vi "Main.vi"() -> ()   [LabVIEW 2017]
doc: "Use this template to build a user interface event handler design pattern. Use this pattern for dialog boxes and other user interfaces. You also can create and execute user-defined events that the VI can handle the same way as user interface events."
uses:
  <vilib>/Utility/NIReport.llb/HTML Report Image Alignment.ctl
  <vilib>/Utility/NIReport.llb/image depth.ctl
  <vilib>/addons/database/Connection.llb/DB Tools Open Connec (Path).vi
  <vilib>/addons/database/Auxilliary.llb/DB Tools Format Datetime String (Time Stamp).vi
  GLOBAL/auto.vi
  <vilib>/Utility/NIReport.llb/Append Report Text (str wrap).vi
  <vilib>/Utility/NIReport.llb/NI_report.lvclass
  <vilib>/addons/database/NI_Database_API.lvlib
  <vilib>/Utility/NIReport.llb/NI_ReportGenerationCore.lvlib
panel:
  out "resulting string":path
  in  "import state 3":bool
  out "User Name":string
  out "time taken in sec":dbl
  out "Peak_valley_point":ext[](array[numeric])
  out "data size":i32
  out "A*C":bool
  out "L/Min":bool
  out "BAR":bool
  out "Min Peak/Min":dbl
  out "Max Valley/Min":dbl
  out "Status bar":string
  in  "import state 2":bool
  out "SELECTED RECIPE":string
  out "BARCODE_FOUND":bool
  out "DB CONN":bool
  in  "Graph":bool
  out "table":string[][](table)
  out "GRAPH":cluster{timestamp[], ext[]}[](graph)
  out "TEST RESULT":bool
  in  "BARCODE":string
  out "SELECTED FILE PATH":path
  in  "Import File":bool
  in  "SELECT MEASURED FILE":i32(listbox)
  out "error out":errorcluster
  in  "File Name":string
  in  "Report Files Folder":path
  in  "Convert":bool
  in  "BROWSE FILE FOLDER":path
  in  "stop":bool
  # "Main"
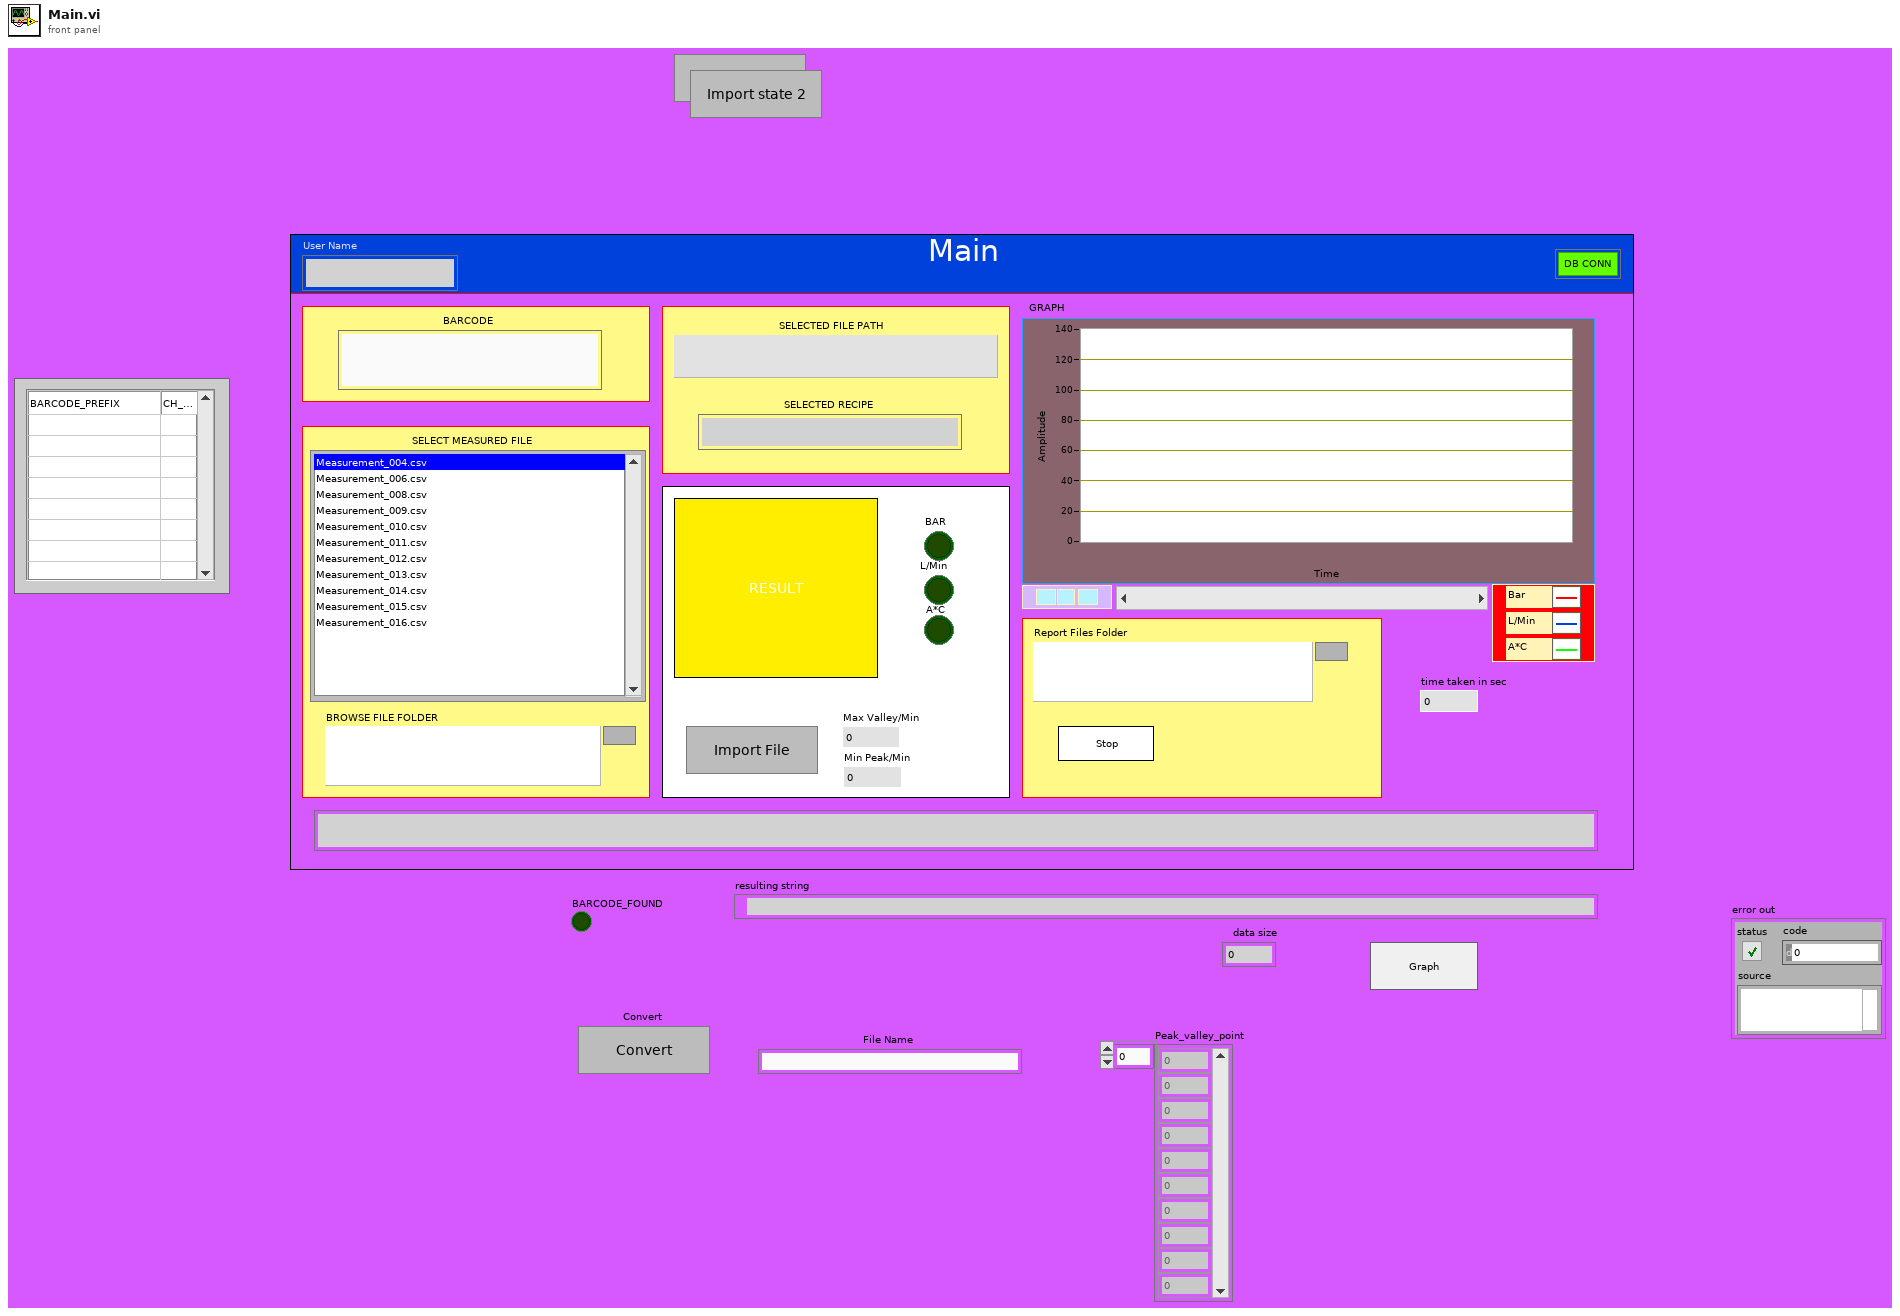
[diagram p1: front panel]
types:
  T1 = cluster{"Files":string[], "Browse File":path, "TIMEOUT":i32, "GRAPH":cluster{timestamp[], ext[]}[], "CHL 1":cluster{"chl1 MIN":dbl, "chl1 MAX":dbl, "chl1 thrshold":dbl}, "CHL 2":cluster{"chl2 MIN":dbl, "chl2 MAX":dbl, "chl2 thrshold":dbl}, "CHL 3":cluster{"chl3 MIN":dbl, "chl3 MAX":dbl, "chl3 thrshold":dbl}, "Report File":path, "Data_to_report":cluster{"date/time string":string, "User Name":string, "BARCODE":string, "SELECTED RECIPE":string, "Rst":string}}
  T2 = typedef "NI_Database_API.lvlib/Conn ObjectReference.ctl" = refnum<k1>
  T3 = enum32{"Invalid", "Standard", "Closed", "Hidden", "Minimized", "Maximized"}
  T4 = cluster{"position (excel)":cluster{"row":i32, "column":i32}, "name (excel)":string, "bookmark (word)":string}
  T5 = cluster{"position (Excel)":cluster{"row":i32, "column":i32}, "name (Excel)":string, "bookmark (Word)":string}
  T6 = typedef "NI_ReportGenerationCore.lvlib/HTML Report Image Alignment.ctl" = enum16{"(default)", "LEFT", "RIGHT", "TOP", "TEXTTOP", "MIDDLE", "ABSMIDDLE", "BASELINE", "BOTTOM", "ABSBOTTOM"}
  T7 = enum16{"Standard Report", "HTML", "Word", "Excel"}
  T8 = enum16{"maximized", "minimized", "normal", "no change"}
  T9 = cluster{"chl2 MIN":dbl, "chl2 MAX":dbl, "chl2 thrshold":dbl}
  T10 = cluster{"chl1 MIN":dbl, "chl1 MAX":dbl, "chl1 thrshold":dbl}
  T11 = cluster{"chl3 MIN":dbl, "chl3 MAX":dbl, "chl3 thrshold":dbl}
  T12 = cluster{"date/time string":string, "User Name":string, "BARCODE":string, "SELECTED RECIPE":string, "Rst":string}
  T13 = typedef "NI_ReportGenerationCore.lvlib/image depth.ctl" = u16
  T14 = enum32{"invalid app kind", "Development System", "Run Time System", "Student Edition", "Embedded LabVIEW", "Evaluation", "Custom"}
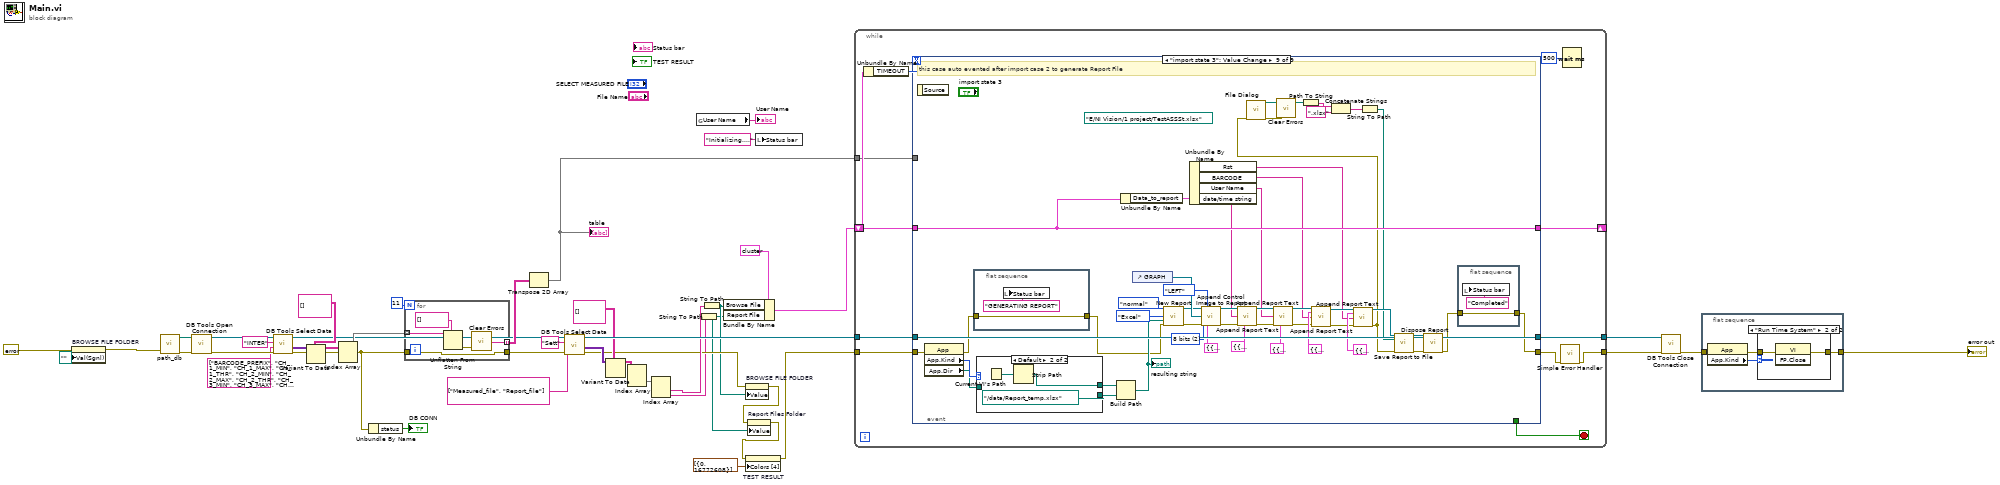
[diagram p0: block diagram]
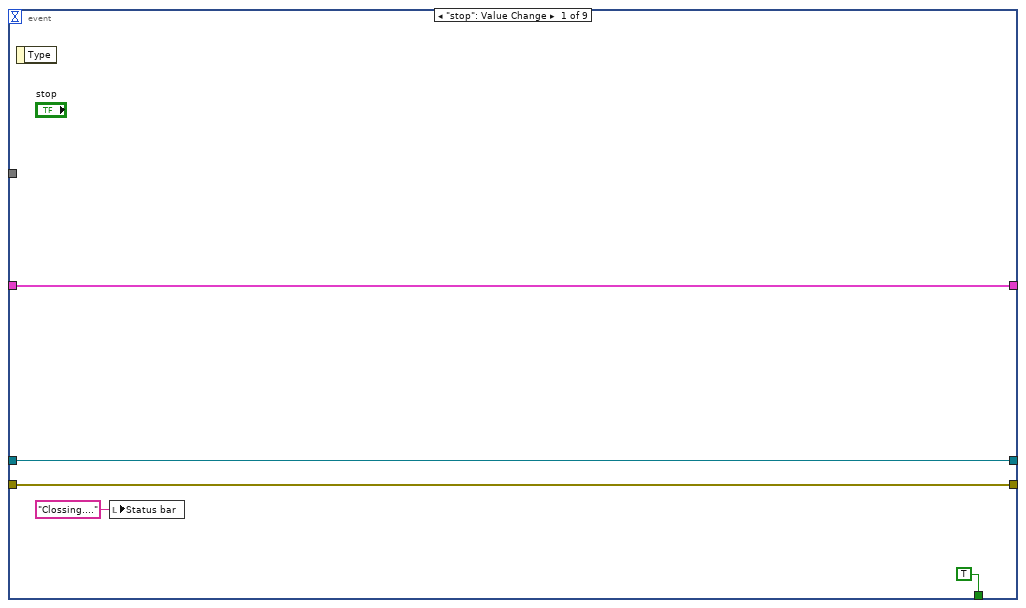
[diagram p3: hidden frame]
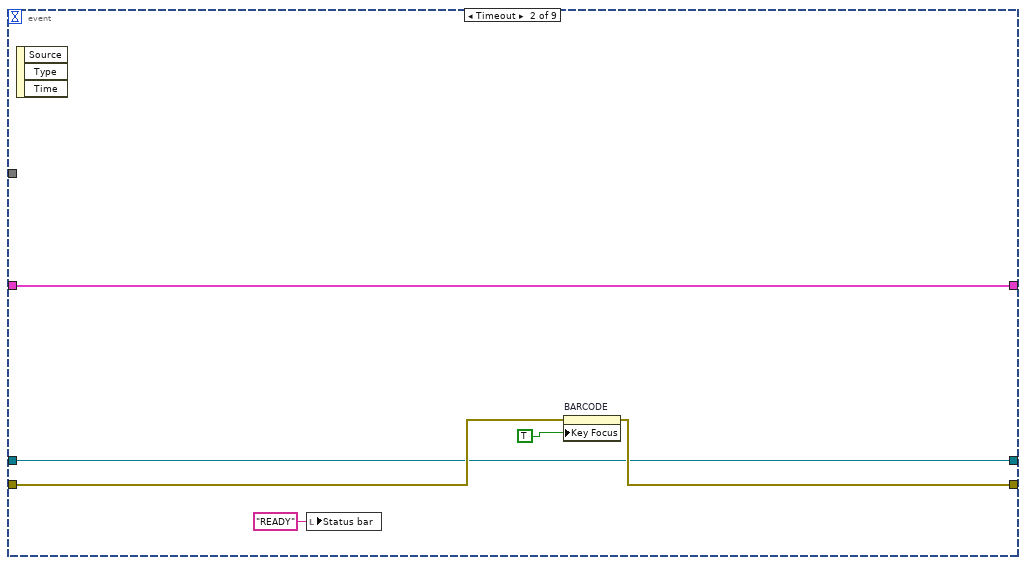
[diagram p4: hidden frame]
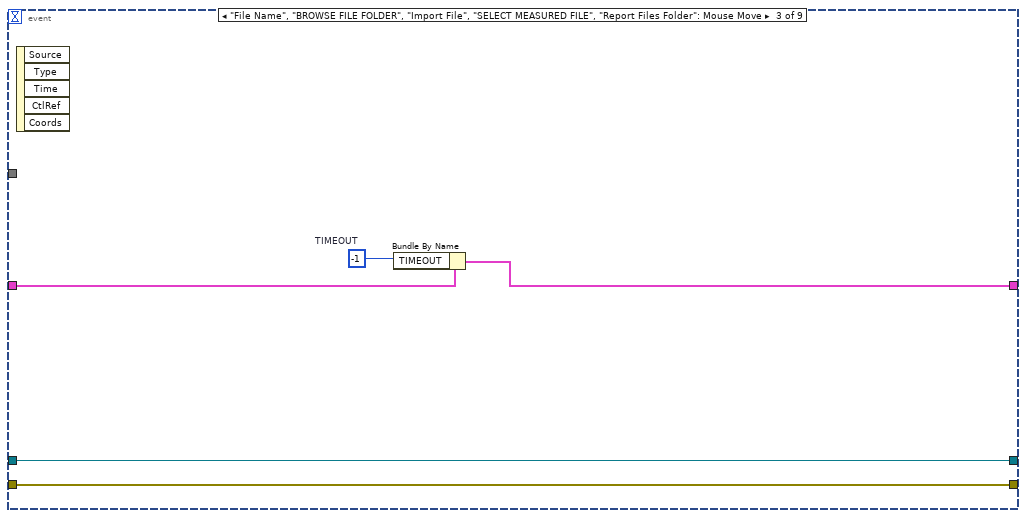
[diagram p5: hidden frame]
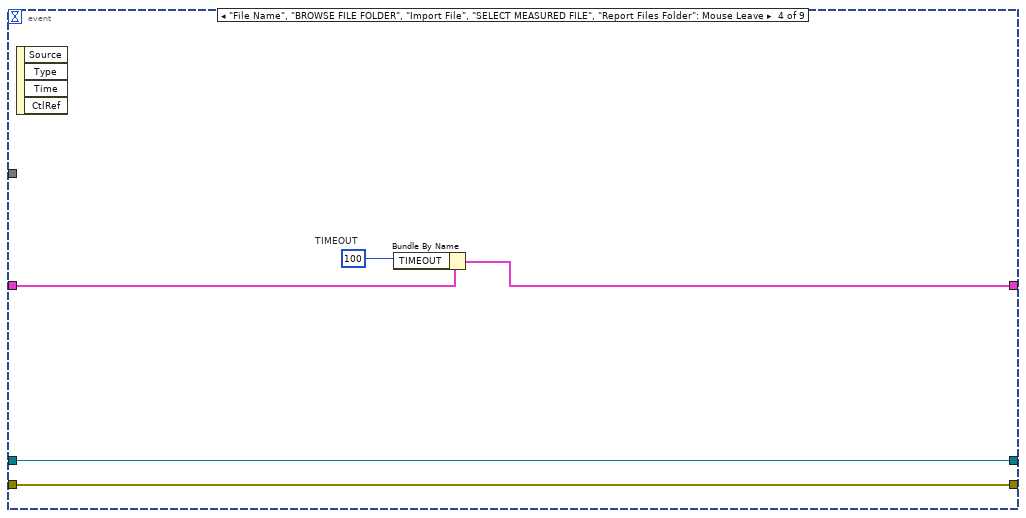
[diagram p6: hidden frame]
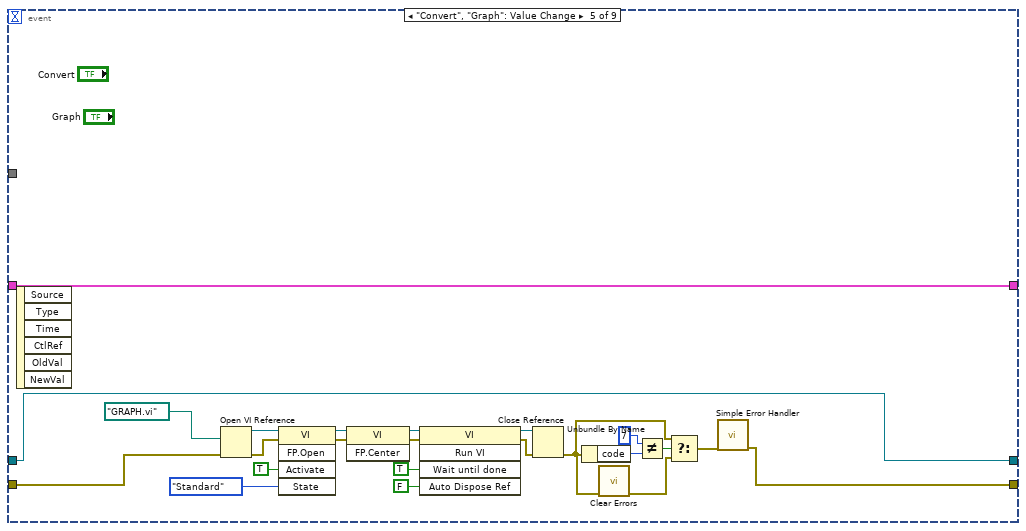
[diagram p7: hidden frame]
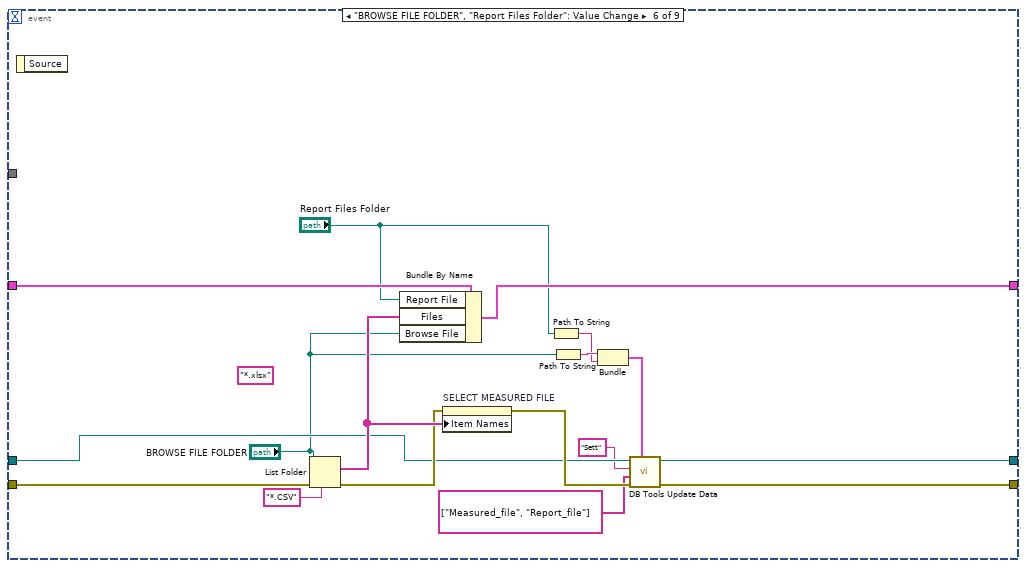
[diagram p8: hidden frame]
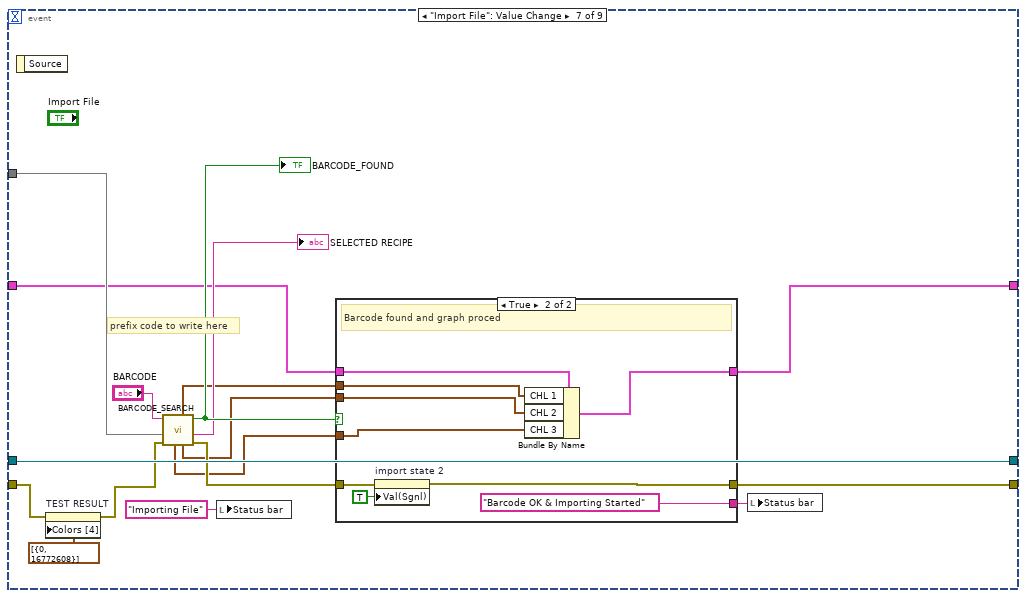
[diagram p9: hidden frame]
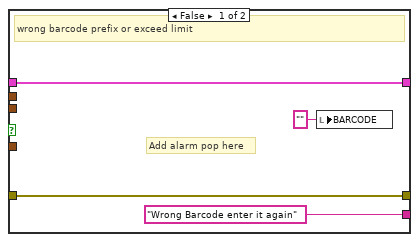
[diagram p10: hidden frame]
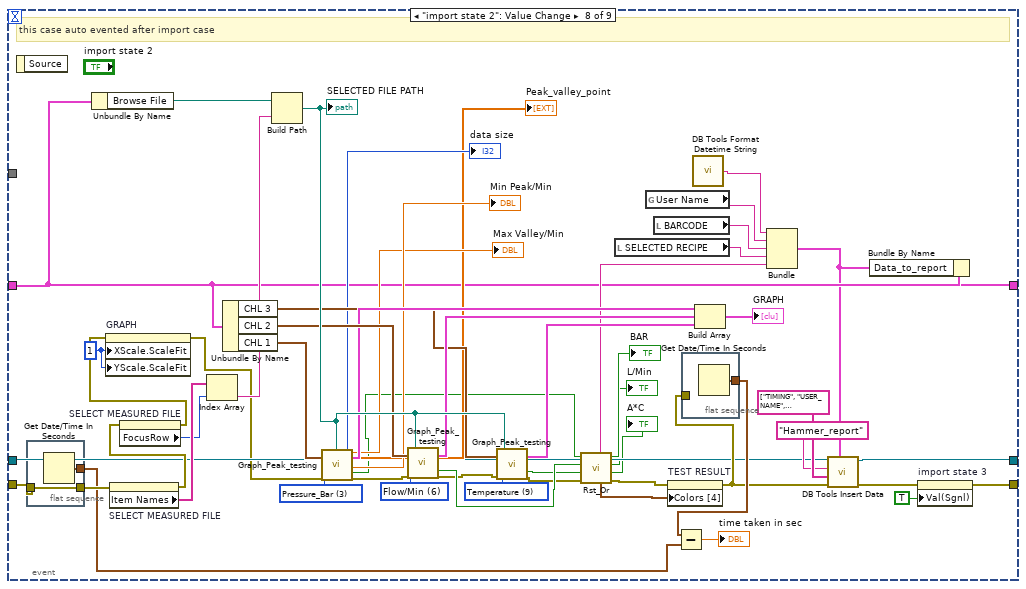
[diagram p11: hidden frame]
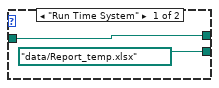
[diagram p12: hidden frame]
diagram:
  n1 = property on="BROWSE FILE FOLDER" class="Path"(error in=errorcluster {"status"=FALSE, "code"=0, "source"=""} ("error out 2"), "Val(Sgnl)"=path "" ("BROWSE FILE FOLDER")) -> (error out=w13:errorcluster)  [unwired: 1 in, 1 out]
  n2 = call "path_db.vi"("error in"=w13) -> ("error out"=w38:errorcluster, "resulting string"=w37:path)  [unwired: 9 in]
  n3 = call-poly <vilib>:"DB Tools Open Connection.vi"("error in (no error)"=w38, "connection information"=w37) -> ("error out"=w43:errorcluster, "connection reference"=w44:T2)  [unwired: 6 in]
  n4 = call <vilib>:"DB Tools Select Data.vi"("error in (no error)"=w43, "columns"=string[] ["BARCODE_PREFIX", "CH_1_MIN", "CH_1_MAX", "CH_1_THR", "CH_2_MIN", "CH_2_MAX", "CH_2_THR", "CH_3_MIN", "CH_3_MAX", "CH_3_THR", "RECIPE_NAME"], "table"="INTER", "connection reference"=w44) -> ("error out"=w31:errorcluster, "data"=w40:variant[][], "connection reference out"=w26:T2)  [unwired: 2 in]
  n5 = Variant To Data(type=string[][] [], Variant=w40) -> (data=w39:string[][])  [unwired: 1 in, 1 out]
  n6 = Index Array(array=w39) -> (element=w34:string[])  [unwired: 2 in]
  n7 = Unbundle By Name(w31) -> ("status"=→"DB CONN":bool)
  n8 = for {
    N: 11 -> [_]
    tunnel: w34 -> [w48] mode=indexing
    tunnel: [w46] -> w33 mode=indexing
    tunnel: w31 -> [w45]
    tunnel: [w45] -> w27
    n9 = Unflatten From String(type=string[] [], binary string=w48) -> (value=w46:string[], error out=w49:errorcluster)  [unwired: 3 in, 1 out]
    n10 = call <vilib>:"Clear Errors.vi"("error in (no error)"=w49) -> ()  [unwired: 5 in, 2 out]
  }
  n11 = Transpose 2D Array(2D array=w33) -> (transposed array=w11:string[][])
  "table" <- w11
  n12 = call <vilib>:"DB Tools Select Data.vi"("error in (no error)"=w27, "columns"=string[] ["Measured_file", "Report_file"], "table"="Sett", "connection reference"=w26) -> ("error out"=w16:errorcluster, "data"=w24:variant[][], "connection reference out"=w25:T2)  [unwired: 2 in]
  n13 = Variant To Data(type=string[][] [], Variant=w24) -> (data=w22:string[][])  [unwired: 1 in, 1 out]
  n14 = Index Array(array=w22) -> (element=w18:string[])  [unwired: 2 in]
  n15 = Index Array(array=w18) -> (element #1=w17:string, element #2=w10:string)  [unwired: 2 in]
  n16 = global read "auto.vi" "User Name"() -> (→"User Name":string)
  n17 = String To Path(string=w10) -> (path=w9:path)
  n18 = String To Path(string=w17) -> (path=w15:path)
  n19 = Bundle By Name(cluster=T1 {"Files"=[], "Browse File"=path "", "TIMEOUT"=100, "GRAPH"=[{array[68443 elements], array[68443 elements]}, {array[68363 elements], array[68363 elements]}, {array[40500 elements], array[40500 elements]}], "CHL 1"={"chl1 MIN"=110.0, "chl1 MAX"=130.0, "chl1 thrshold"=120.0}, "CHL 2"={"chl2 MIN"=33.0, "chl2 MAX"=35.0, "chl2 thrshold"=25.0}, "CHL 3"={"chl3 MIN"=20.0, "chl3 MAX"=30.0, "chl3 thrshold"=34.0}, "Report File"=path "", "Data_to_report"={"date/time string"="", "User Name"="", "BARCODE"="", "SELECTED RECIPE"="", "Rst"=""}}, "Browse File"=w15, "Report File"=w9) -> (w19:T1)
  n20 = property on="BROWSE FILE FOLDER" class="Path"(error in=w16, "Value"=w15) -> (error out=w8:errorcluster)  [unwired: 1 in, 1 out]
  n21 = property on="Report Files Folder" class="Path"(error in=w8, "Value"=w9) -> (error out=w7:errorcluster)  [unwired: 1 in, 1 out]
  n22 = property on="TEST RESULT" class="Bool"(error in=w7, "Colors [4]"=cluster{u32, u32}[] [{0, 16772608}]) -> (error out=w1:errorcluster)  [unwired: 1 in, 1 out]
  n23 = local write "Status bar"("Initializing...." ("Status bar")) -> ()
  n24 = while {
    tunnel: w1 -> [w58]
    tunnel: [w50] -> w30
    shift-right: [w57] -> _
    shift-left: w19 -> [w55]
    tunnel: w25 -> [w53]
    tunnel: [w54] -> w29
    tunnel: w11 -> [w52]
    stop <- w60 stop-if-true
    n25 = Unbundle By Name(w55) -> ("TIMEOUT"=w56:i32)
    n26 = event shown="[8] \"import state 3\": Value Change" {
      selector: _ -> [_ _ _ _ _ _ _ _ _]
      dyn-events: _ -> [_ _ _ _ _ _ _ _ _]
      timeout: w56 -> [_ _ _ _ _ _ _ _ _]
      tunnel: [TRUE _ _ _ _ _ _ _ _] -> w60
      tunnel: w58 -> [w64 w69 w76 w81 w84 w121 w125 w187 w251]
      tunnel: [w64 w68 w76 w81 w83 w114 w135 w162 w218] -> w51
      tunnel: w55 -> [w65 w71 w75 w80 w104 w120 w131 w160 w239]
      tunnel: [w65 w71 w74 w79 w104 w119 w130 w159 w239] -> w57
      tunnel: [w62 w67 w72 w77 w82 w112 w138 w178 w256] -> w54
      tunnel: w53 -> [w62 w67 w72 w77 w82 w113 w138 w179 w256]
      tunnel: w52 -> [_ _ _ _ _ _ w132 _ _]
      event "stop": Value Change {
        n27 = event-data() -> ()  [unwired: 1 in, 1 out]
        n28 = local write "Status bar"("Clossing...." ("Status bar")) -> ()
      }
      event Timeout {
        n29 = event-data() -> ()  [unwired: 1 in, 3 out]
        n30 = local write "Status bar"("READY" ("Status bar")) -> ()
        n31 = property on="BARCODE" class="Str"(error in=w69, "Key Focus"=TRUE) -> (error out=w68:errorcluster)  [unwired: 1 in, 1 out]
      }
      event "File Name", "BROWSE FILE FOLDER", "Import File", "SELECT MEASURED FILE", "Report Files Folder": Mouse Move {
        w73 = -1  # TIMEOUT
        n32 = event-data() -> ()  [unwired: 1 in, 5 out]
        n33 = Bundle By Name(cluster=w75, "TIMEOUT"=w73) -> (w74:T1)
      }
      event "File Name", "BROWSE FILE FOLDER", "Import File", "SELECT MEASURED FILE", "Report Files Folder": Mouse Leave {
        w78 = 100  # TIMEOUT
        n34 = event-data() -> ()  [unwired: 1 in, 4 out]
        n35 = Bundle By Name(cluster=w80, "TIMEOUT"=w78) -> (w79:T1)
      }
      event "Convert", "Graph": Value Change {
        n36 = event-data() -> ()  [unwired: 1 in, 6 out]
        n37 = Open VI Reference(vi path=path "GRAPH.vi", error in (no error)=w84) -> (vi reference=w91:refnum<vi>, error out=w103:errorcluster)  [unwired: 4 in]
        n38 = invoke class="VI" method="FP.Open"(reference=w91, error in=w103, "Activate"=TRUE ("Activate?"), "State"=T3."Standard") -> (reference out=w102:refnum<vi>, error out=w97:errorcluster)  [unwired: 1 in, 3 out]
        n39 = invoke class="VI" method="FP.Center"(reference=w102, error in=w97) -> (reference out=w98:refnum<vi>, error out=w99:errorcluster)  [unwired: 1 in, 1 out]
        n40 = invoke class="VI" method="Run VI"(reference=w98, error in=w99, "Wait until done"=TRUE ("Wait Until Done"), "Auto Dispose Ref"=FALSE ("Auto Dispose Reference")) -> (reference out=w100:refnum<vi>, error out=w101:errorcluster)  [unwired: 1 in, 3 out]
        n41 = Close Reference(reference=w100, error in (no error)=w101) -> (error out=w92:errorcluster)
        n42 = Unbundle By Name(w92) -> ("code"=w96:i32)
        n43 = call <vilib>:"Clear Errors.vi"("error in (no error)"=w92) -> ("error out"=w94:errorcluster)  [unwired: 5 in, 1 out]
        n44 = Not Equal?(x=7, y=w96) -> (x != y?=w95:bool)
        n45 = Select(t=w92, s=w95, f=w94) -> (s? t:f=w93:errorcluster)
        n46 = call <vilib>:"Simple Error Handler.vi"("error in (no error)"=w93) -> ("error out"=w83:errorcluster)  [unwired: 4 in, 4 out]
      }
      event "BROWSE FILE FOLDER", "Report Files Folder": Value Change {
        (unwired) "*.xlsx" ("pattern")
        n47 = event-data() -> ()  [unwired: 1 in, 1 out]
        n48 = List Folder(path="BROWSE FILE FOLDER", pattern="*.CSV", error in=w121) -> (filenames=w117:string[], error out=w116:errorcluster)  [unwired: 1 in, 2 out]
        n49 = Bundle By Name(cluster=w120, "Report File"="Report Files Folder", "Files"=w117, "Browse File"="BROWSE FILE FOLDER") -> (w119:T1)
        n50 = property on="SELECT MEASURED FILE" class="LstBox (strict)"(error in=w116, "Item Names"=w117) -> (error out=w115:errorcluster)  [unwired: 1 in, 1 out]
        n51 = Path To String(path="Report Files Folder") -> (string=w106:string)
        n52 = Path To String(path="BROWSE FILE FOLDER") -> (string=w108:string)
        n53 = Bundle(w108, w106) -> (w111:cluster{string, string})  [unwired: 1 in]
        n54 = call <vilib>:"DB Tools Update Data.vi"("data"=w111, "error in (no error)"=w115, "columns"=string[] ["Measured_file", "Report_file"], "table"="Sett", "connection reference"=w113) -> ("error out"=w114:errorcluster, "connection reference out"=w112:T2)  [unwired: 5 in]
      }
      event "Import File": Value Change {
        # "prefix code to write here"
        n55 = event-data() -> ()  [unwired: 1 in, 1 out]
        n56 = property on="TEST RESULT" class="Bool"(error in=w125, "Colors [4]"=cluster{u32, u32}[] [{0, 16772608}]) -> (error out=w124:errorcluster)  [unwired: 1 in, 1 out]
        n57 = call "BARCODE_SEARCH.vi"("error in"=w124, "BARCODE_TABLE"=w132, "BARCODE_TO_SEARCH"="BARCODE") -> ("error out"=w136:errorcluster, "Recipe name"=→"SELECTED RECIPE":string, "BARCODE_FOUND"=w134:bool, "CHL 2"=w128:T9, "CHL 1"=w129:T10, "CHL 3"=w127:T11)  [unwired: 2 in, 1 out]
        "BARCODE_FOUND" <- w134
        n58 = local write "Status bar"("Importing File" ("Status bar")) -> ()
        n59 = case shown="True" w134 {
          tunnel: [w142 w149] -> w135
          tunnel: w136 -> [w142 w150]
          tunnel: [w141 w147] -> w130
          tunnel: w131 -> [w141 w148]
          tunnel: w129 -> [_ w146]
          tunnel: w128 -> [_ w145]
          tunnel: w127 -> [_ w144]
          tunnel: ["Wrong Barcode enter it again" ("Status bar") "Barcode OK & Importing Started" ("Status bar")] -> w122
          frame False {
            # "Add alarm pop here"
            # "wrong barcode prefix or exceed limit"
            n60 = local write "BARCODE"("" ("BARCODE")) -> ()
          }
          frame True {
            # "Barcode found and graph proced"
            n61 = property on="import state 2" class="Bool (strict)"(error in=w150, "Val(Sgnl)"=TRUE) -> (error out=w149:errorcluster)  [unwired: 1 in, 1 out]
            n62 = Bundle By Name(cluster=w148, "CHL 1"=w146, "CHL 2"=w145, "CHL 3"=w144) -> (w147:T1)
          }
        }
        n63 = local write "Status bar"(w122) -> ()
      }
      event "import state 2": Value Change {
        w156 = u8 1 ("X Scale.Scale Fit")
        w173 = u16 9 items=["Temperature"=9, "Flow/Min"=6, "Pressure_Bar"=3] ("Channel Select")
        w197 = u16 6 items=["BPM"=9, "Flow/Min"=6, "Pressure_Bar"=3] ("Channel Select")
        w198 = u16 3 items=["BPM"=9, "Flow/Min"=6, "Pressure_Bar"=3] ("Channel Select")
        # "this case auto evented after import case"
        n64 = event-data() -> ()  [unwired: 1 in, 1 out]
        n65 = flat-sequence {
          tunnel: [w208] -> w184
          tunnel: [w207] -> w186
          tunnel: w187 -> [w207]
          frame #0 {
            n66 = Get Date/Time In Seconds() -> (seconds since 1Jan1904=w208:timestamp)
          }
        }
        n67 = Unbundle By Name(w160) -> ("Browse File"=w204:path)
        n68 = property on="SELECT MEASURED FILE" class="LstBox (strict)"(error in=w186) -> (error out=w202:errorcluster, "Item Names"=w206:string[])  [unwired: 1 in, 1 out]
        n69 = property on="SELECT MEASURED FILE" class="LstBox (strict)"(error in=w202) -> (error out=w157:errorcluster, "FocusRow"=w205:i32)  [unwired: 1 in, 1 out]
        n70 = property on="GRAPH" class="XYGraph (strict)"(error in=w157, "XScale.ScaleFit"=w156, "YScale.ScaleFit"=w156) -> (error out=w155:errorcluster)  [unwired: 1 in, 1 out]
        n71 = Index Array(array=w206, index=w205) -> (element=w203:string)
        n72 = Unbundle By Name(w160) -> ("CHL 3"=w193:T11, "CHL 2"=w199:T9, "CHL 1"=w192:T10)
        n73 = Build Path(base path=w204, name or relative path=w203) -> (appended path=w201:path)
        "SELECTED FILE PATH" <- w201
        n74 = call "Graph_Peak_testing.vi"("Channel Select"=w198, "CHL"=w192, "error in"=w155, "CSV file path"=w201) -> ("size(s)"=→"data size":i32, "Peak_valley_point"=→"Peak_valley_point":ext[], "Max Valley/Min"=→"Max Valley/Min":dbl, "XY Graph 2"=w194:cluster{timestamp[], ext[]}, "Min Valley/Min"=→"Min Peak/Min":dbl, "Peak or Valley Fail"=w169:bool, "error out"=w154:errorcluster)  [unwired: 5 in, 4 out]
        n75 = call "Graph_Peak_testing.vi"("Channel Select"=w197, "CHL"=w199, "error in"=w154, "CSV file path"=w201) -> ("XY Graph 2"=w195:cluster{timestamp[], ext[]}, "Peak or Valley Fail"=w168:bool, "error out"=w153:errorcluster)  [unwired: 5 in, 8 out]
        n76 = call "Graph_Peak_testing.vi"("Channel Select"=w173, "CHL"=w193, "error in"=w153, "CSV file path"=w201) -> ("XY Graph 2"=w196:cluster{timestamp[], ext[]}, "Peak or Valley Fail"=w167:bool, "error out"=w152:errorcluster)  [unwired: 5 in, 8 out]
        n77 = call "Rst_Or.vi"("error In"=w152, "A*C rst"=w167, "L/Min rst"=w168, "BAR rst"=w169) -> ("error out"=w172:errorcluster, "A*C"=→"A*C":bool, "L/Min"=→"L/Min":bool, "BAR"=→"BAR":bool, "Rst ind Color"=w171:cluster{u32, u32}[], "Rst"=w170:string)  [unwired: 2 in]
        n78 = local read "SELECTED RECIPE"() -> (w177:string)
        n79 = global read "auto.vi" "User Name"() -> (w174:string)
        n80 = local read "BARCODE"() -> (w176:string)
        n81 = property on="TEST RESULT" class="Bool"(error in=w172, "Colors [4]"=w171) -> (error out=w180:errorcluster)  [unwired: 1 in, 1 out]
        n82 = Subtract(x=w185, y=w184) -> (x-y=→"time taken in sec":dbl)
        n83 = flat-sequence {
          tunnel: [w209] -> w185
          tunnel: w180 -> [_]
          frame #0 {
            n84 = Get Date/Time In Seconds() -> (seconds since 1Jan1904=w209:timestamp)
          }
        }
        n85 = call-poly <vilib>:"DB Tools Format Datetime String.vi"() -> ("date/time string"=w175:string)  [unwired: 1 in]
        n86 = Build Array(w194, w195, w196) -> (→"GRAPH":cluster{timestamp[], ext[]}[])
        n87 = Bundle("date/time string"=w175, "User Name"=w174, "BARCODE"=w176, "SELECTED RECIPE"=w177, "Rst"=w170) -> (w158:T12)  [unwired: 1 in]
        n88 = call <vilib>:"DB Tools Insert Data.vi"("data"=w158, "error in (no error)"=w180, "columns"=string[] ["TIMING", "USER_NAME", "BARCODE", "RECIPE_NAME", "RST_STATUS"], "table"="Hammer_report", "connection reference"=w179) -> ("error out"=w163:errorcluster, "connection reference out"=w178:T2)  [unwired: 5 in]
        n89 = Bundle By Name(cluster=w160, "Data_to_report"=w158) -> (w159:T1)
        n90 = property on="import state 3" class="Bool (strict)"(error in=w163, "Val(Sgnl)"=TRUE) -> (error out=w162:errorcluster)  [unwired: 1 in, 1 out]
      }
      event "import state 3": Value Change {
        (unwired) path "E:/NI Vision/1 project/TestASSSt.xlsx" ("report file path")
        w240 = T13 2 items=["B&W", "4 bits", "8 bits", "24 bits"] ("image depth")
        # "this case auto evented after import case 2 to generate Report File"
        n91 = event-data() -> ()  [unwired: 1 in, 1 out]
        n92 = property class="App"(error in=w251) -> (error out=w220:errorcluster, "App.Kind"=w255:T14, "App.Dir"=w254:path)  [unwired: 1 in, 1 out]
        n93 = flat-sequence {
          tunnel: w220 -> [w259]
          tunnel: [w259] -> w219
          frame #0 {
            n94 = local write "Status bar"("GENERATING REPORT" ("Status bar")) -> ()
          }
        }
        n95 = case shown="Default" w255 {
          tunnel: w254 -> [w262 _]
          tunnel: [path "data/Report_temp.xlsx" ("path") path "../data/Report_temp.xlsx" ("path")] -> w253
          tunnel: [w262 w263] -> w252
          frame "Run Time System" {
          }
          frame Default {
            n96 = Current VI's Path() -> (path=w264:path)
            n97 = Strip Path(path=w264) -> (stripped path=w263:path)  [unwired: 1 out]
          }
        }
        n98 = Build Path(base path=w252, name or relative path=w253) -> (appended path=w245:path)
        "resulting string" <- w245
        n99 = Unbundle By Name(w239) -> ("Data_to_report"=w238:T12)
        n100 = control-ref of="GRAPH"() -> (w248:refnum<vi>)
        n101 = call <vilib>:"New Report.vi"("window state (normal)"=T8."normal", "report type"=T7."Excel", "template (empty)"=w245, "error in (no error)"=w219) -> ("report out"=w247:refnum<class "NI_report.lvclass">, "error out"=w246:errorcluster)  [unwired: 10 in]
        n102 = Unbundle By Name(w238) -> ("Rst"=w222:string, "BARCODE"=w226:string, "User Name"=w231:string, "date/time string"=w234:string)
        n103 = call-dynamic "Append Control Image to Report.vi"("report in"=w247, "alignment (default)"=HTML_Report_Image_Alignment."LEFT", "image depth"=w240, "ctrl reference"=w248, "error in (no error)"=w246, "MS Office parameters"=T5 {"position (Excel)"={"row"=14, "column"=0}, "name (Excel)"="", "bookmark (Word)"=""}) -> ("report out"=w237:refnum<class "NI_report.lvclass">, "error out"=w236:errorcluster)  [unwired: 6 in, 2 out]
        n104 = call-poly <vilib>:"Append Report Text.vi"("report in"=w237, "MS Office parameters"=T5 {"position (Excel)"={"row"=2, "column"=1}, "name (Excel)"="", "bookmark (Word)"=""}, "text"=w234, "error in (no error)"=w236) -> ("report out"=w233:refnum<class "NI_report.lvclass">, "error out"=w232:errorcluster)  [unwired: 8 in, 2 out]
        n105 = call-poly <vilib>:"Append Report Text.vi"("report in"=w233, "MS Office parameters"=T4 {"position (excel)"={"row"=3, "column"=1}, "name (excel)"="", "bookmark (word)"=""}, "text"=w231, "error in (no error)"=w232) -> ("report out"=w227:refnum<class "NI_report.lvclass">, "error out"=w228:errorcluster)  [unwired: 8 in, 2 out]
        n106 = call-poly <vilib>:"Append Report Text.vi"("report in"=w227, "MS Office parameters"=T4 {"position (excel)"={"row"=2, "column"=5}, "name (excel)"="", "bookmark (word)"=""}, "text"=w226, "error in (no error)"=w228) -> ("report out"=w223:refnum<class "NI_report.lvclass">, "error out"=w224:errorcluster)  [unwired: 8 in, 2 out]
        n107 = call-poly <vilib>:"Append Report Text.vi"("report in"=w223, "MS Office parameters"=T4 {"position (excel)"={"row"=12, "column"=1}, "name (excel)"="", "bookmark (word)"=""}, "text"=w222, "error in (no error)"=w224) -> ("report out"=w221:refnum<class "NI_report.lvclass">, "error out"=w210:errorcluster)  [unwired: 8 in, 2 out]
        n108 = call "File Dialog"("error in"=w210) -> ("selected path"=w216:path, "error out"=w211:errorcluster)  [unwired: 11 in, 2 out]
        n109 = call <vilib>:"Clear Errors.vi"("error in (no error)"=w211) -> ()  [unwired: 5 in, 2 out]
        n110 = Path To String(path=w216) -> (string=w215:string)
        n111 = Concatenate Strings(w215, ".xlsx" ("string")) -> (w213:string)
        n112 = String To Path(string=w213) -> (path=w212:path)
        n113 = call-dynamic "Save Report to File.vi"("report in"=w221, "report file path"=w212, "error in (no error)"=w210) -> ("report out"=w250:refnum<class "NI_report.lvclass">, "error out"=w249:errorcluster)  [unwired: 11 in]
        n114 = call-dynamic "Dispose Report.vi"("report in"=w250, "error in (no error)"=w249) -> ("error out"=w217:errorcluster)  [unwired: 13 in]
        n115 = flat-sequence {
          tunnel: w217 -> [w257]
          tunnel: [w257] -> w218
          frame #0 {
            n116 = local write "Status bar"("Completed" ("Status bar")) -> ()
          }
        }
      }
    }
    n117 = call <vilib>:"Simple Error Handler.vi"("error in (no error)"=w51) -> ("error out"=w50:errorcluster)  [unwired: 4 in, 4 out]
    n118 = Wait (ms)(milliseconds to wait=u32 500) -> ()  [unwired: 1 out]
  }
  n119 = call <vilib>:"DB Tools Close Connection.vi"("error in (no error)"=w30, "connection reference"=w29) -> ("error out"=w3:errorcluster)  [unwired: 5 in]
  n120 = flat-sequence {
    tunnel: [w266] -> w2
    tunnel: w3 -> [w267]
    frame #0 {
      n121 = property class="App"(error in=w267) -> (error out=w268:errorcluster, "App.Kind"=w269:T14)  [unwired: 1 in, 1 out]
      n122 = case shown="\"Run Time System\"" w269 {
        tunnel: w268 -> [w270 w272]
        tunnel: [w270 w271] -> w266
        frame Default {
        }
        frame "Run Time System" {
          n123 = invoke class="VI" method="FP.Close"(error in=w272) -> (error out=w271:errorcluster)  [unwired: 2 in, 2 out]
        }
      }
    }
  }
  "error out" <- w2
